vi "Specify Delete Action.vi"(11 "Endpoint in":refnum<class "Endpoint.lvclass">) -> (2 "Delete action":string, 3 "Endpoint out":refnum<class "Endpoint.lvclass">)   [LabVIEW 2015, in "NI_AWS_SNS.lvlib" / "Endpoint.lvclass"]
uses:
  Endpoint.lvclass
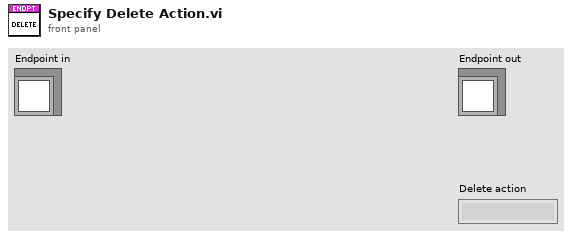
[diagram p1: front panel]
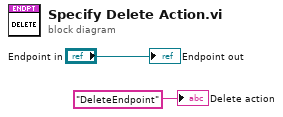
[diagram p0: block diagram]
diagram:
  "Endpoint out" <- "Endpoint in"
  "Delete action" <- "DeleteEndpoint" ("value")
